vi "Read Waveform Segment (DBL).vi"(8 "error in (no error)":errorcluster, 10 "Wfm Segment":T1, 11 "Waveform Buffer in":refnum<class "Waveform Buffer.lvclass">) -> (0 "error out":errorcluster, 2 "Data":dbl[](array[numeric]), 3 "Waveform Buffer out":refnum<class "Waveform Buffer.lvclass">)   [LabVIEW 2015, in "Waveform Data Logger Engine.lvlib" / "Waveform Buffer.lvclass"]
uses:
  Waveform Buffer.lvclass
  Wfm Segment.ctl
  Data Point.ctl
  Waveform Buffer.lvclass/Waveform Buffer.ctl
  DBL Waveform Buffer/DBL Waveform Buffer.lvclass
  DBL Waveform Buffer/DBL Waveform Buffer.lvclass/DBL Waveform Buffer.ctl
  Get Buffer Length.vi
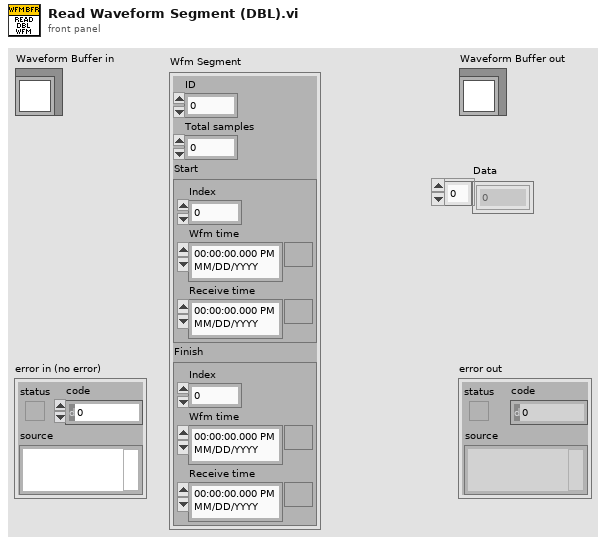
[diagram p1: front panel]
types:
  T1 = typedef "Waveform Data Logger Engine.lvlib/Waveform Buffer.lvclass/Wfm Segment.ctl" = cluster{"ID":u64, "Total samples":i32, "Start":T2, "Finish":T2}
  T2 = typedef "Waveform Data Logger Engine.lvlib/Waveform Buffer.lvclass/Data Point.ctl" = cluster{"Index":i32, "Wfm time":timestamp, "Receive time":timestamp}
  T3 = typedef "Waveform Data Logger Engine.lvlib/Waveform Buffer.lvclass/Buffer Data Type.ctl" = enum16{"Double", "ComplexDouble"}
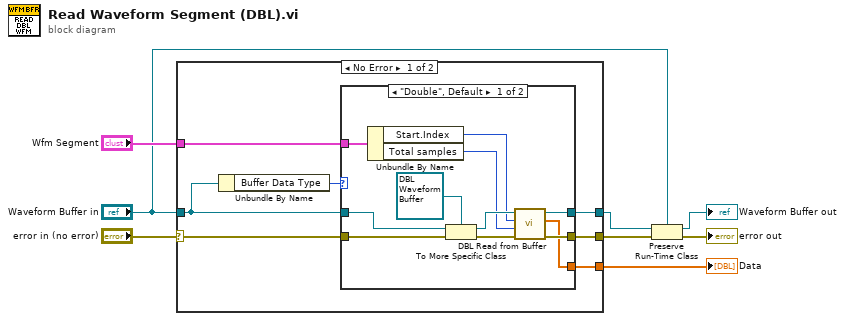
[diagram p0: block diagram]
diagram:
  n1 = case shown="No Error" "error in (no error)" {
    selector: "error in (no error)" -> [w14 w30]
    tunnel: [w13 w30] -> w5
    tunnel: [w12 w29] -> w3
    tunnel: "Waveform Buffer in" -> [w11 w29]
    tunnel: [w10 _] -> w7
    tunnel: "Wfm Segment" -> [w9 _]
    frame No Error {
      n2 = Unbundle By Name(w11) -> ("Buffer Data Type"=w15:T3)
      n3 = case shown="\"Double\", Default" w15 {
        tunnel: w14 -> [w23 w27]
        tunnel: w11 -> [w22 w28]
        tunnel: [w21 w28] -> w12
        tunnel: [w20 w27] -> w13
        tunnel: [w19 _] -> w10
        tunnel: w9 -> [w18 _]
        frame "Double", Default {
          n4 = Unbundle By Name(w18) -> ("Start.Index"=w16:i32, "Total samples"=w17:i32)
          n5 = To More Specific Class(target class=refnum<class "DBL Waveform Buffer.lvclass"> refnum ("Waveform Data Logger Engine.lvlib:DBL Waveform Buffer.lvclass"), reference=w22, error in=w23) -> (specific class reference=w25:refnum<class "DBL Waveform Buffer.lvclass">, error out=w24:errorcluster)
          n6 = call "DBL Read from Buffer.vi"("error in (no error)"=w24, "Length"=w17, "Start Index"=w16, "DBL Waveform Buffer in"=w25) -> ("error out"=w20:errorcluster, "Data"=w19:dbl[], "DBL Waveform Buffer out"=w21:refnum<class "DBL Waveform Buffer.lvclass">)  [unwired: 5 in]
        }
        frame "ComplexDouble" {
        }
      }
    }
    frame Error {
    }
  }
  "Data" <- w7
  n7 = Preserve Run-Time Class(object in=w3, error in=w5, 2:"Waveform Buffer in") -> (object out=→"Waveform Buffer out":refnum<class "Waveform Buffer.lvclass">, error out=→"error out":errorcluster)
